vi "update states from tdms.vi"(8 "error in (no error)":errorcluster, 10 "frot panel referances":T1, 11 "p2p vst in":refnum<class "p2p vst.lvclass">) -> (0 "error out":errorcluster, 2 "tdms file mode":T2=enum."P2P - VST", 3 "p2p vst out":refnum<class "p2p vst.lvclass">)   [LabVIEW 2021, in "p2p vst.lvclass"]
uses:
  p2p vst.lvclass
  p2p vst.lvclass/p2p vst.ctl
  device_type/device_type.lvclass
  pulse_tx_vis/device_mode.ctl
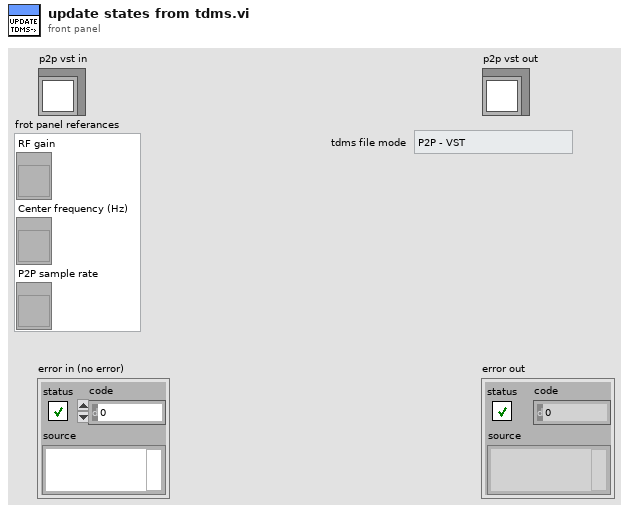
[diagram p1: front panel]
types:
  T1 = cluster{"RF gain ":refnum<vi>, "Center frequency (Hz) ":refnum<vi>, "P2P sample rate":refnum<vi>}
  T2 = typedef "device_mode.ctl" = enum16{"USRP - 180MHz", "5785 - 2*180MHz", "5785 - 3.2GHz", "P2P - VST"}
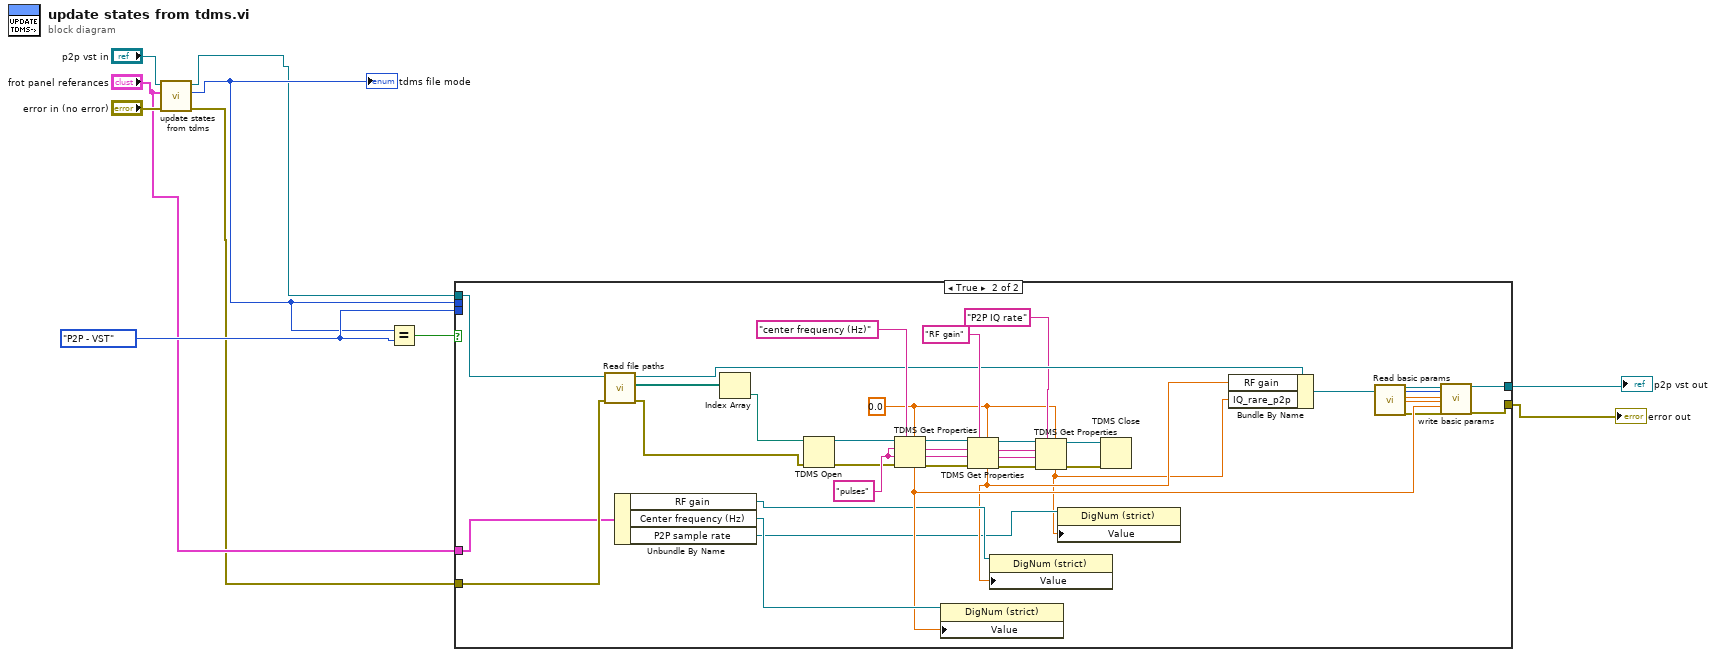
[diagram p0: block diagram]
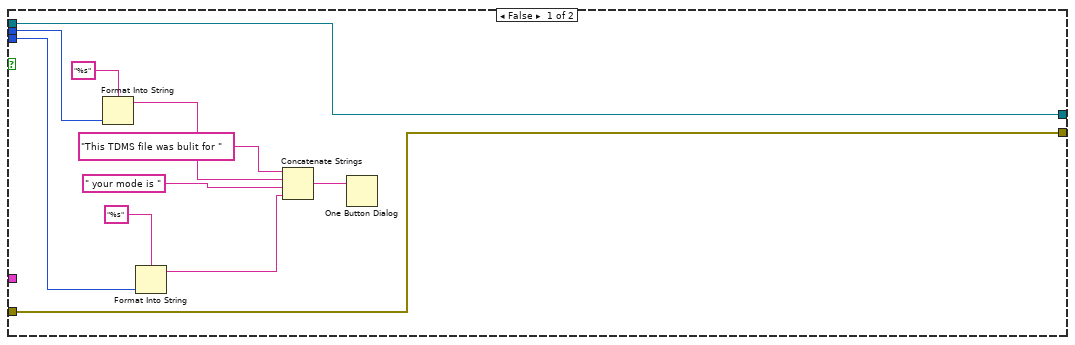
[diagram p2: hidden frame]
diagram:
  w7 = device_mode."P2P - VST" ("Mode")
  n1 = call-parent "update states from tdms.vi"("error in (no error)"="error in (no error)", "frot panel referances"="frot panel referances", "device_type in"="p2p vst in") -> ("error out"=w5:errorcluster, "tdms file mode"=w4:T2, "device_type out"=w3:refnum<class "p2p vst.lvclass">)  [unwired: 6 in]
  "tdms file mode" <- w4
  n2 = Equal?(x=w4, y=w7) -> (x = y?=w8:bool)
  n3 = case shown="True" w8 {
    tunnel: w4 -> [w20 _]
    tunnel: w7 -> [w15 _]
    tunnel: w5 -> [w11 w54]
    tunnel: w3 -> [w12 w52]
    tunnel: "frot panel referances" -> [_ w50]
    tunnel: [w12 w42] -> w1
    tunnel: [w11 w41] -> w2
    frame False {
      n4 = Format Into String(format string="%s", w20) -> (resulting string=w19:string)  [unwired: 2 in, 1 out]
      n5 = Format Into String(format string="%s", w15) -> (resulting string=w14:string)  [unwired: 2 in, 1 out]
      n6 = Concatenate Strings("This TDMS file was bulit for " ("string"), w19, " your mode is " ("string"), w14) -> (w13:string)
      n7 = One Button Dialog(message=w13) -> ()  [unwired: 1 in, 1 out]
    }
    frame True {
      w24 = 0.0
      w59 = "pulses" ("channel name")
      n8 = call-dynamic "Read file paths.vi"("error in (no error)"=w54, "device_type in"=w52) -> ("error out"=w55:errorcluster, "file paths"=w53:path[], "device_type out"=w34:refnum<class "p2p vst.lvclass">)  [unwired: 7 in]
      n9 = Unbundle By Name(w50) -> ("RF gain"=w35:refnum<vi>, "Center frequency (Hz)"=w49:refnum<vi>, "P2P sample rate"=w23:refnum<vi>)
      n10 = Index Array(array=w53) -> (element=w56:path)  [unwired: 1 in]
      n11 = TDMS Open(8:w55, 11:w56) -> (0:w57:errorcluster, 3:w58:refnum<k34>)  [unwired: 5 in]
      n12 = TDMS Get Properties(5:w24, 7:"center frequency (Hz)", 8:w57, 9:w59, 10:w59, 11:w58) -> (0:w37:errorcluster, 1:w38:string, 2:w39:string, 3:w40:refnum<k34>, 4:w44:dbl)  [unwired: 1 out]
      n13 = property class="DigNum (strict)"(reference=w49, "Value"=w44) -> ()  [unwired: 1 in, 2 out]
      n14 = TDMS Get Properties(5:w24, 7:"RF gain", 8:w37, 9:w38, 10:w39, 11:w40) -> (0:w28:errorcluster, 1:w29:string, 2:w30:string, 3:w31:refnum<k34>, 4:w33:dbl)  [unwired: 1 out]
      n15 = property class="DigNum (strict)"(reference=w35, "Value"=w33) -> ()  [unwired: 1 in, 2 out]
      n16 = TDMS Get Properties(5:w24, 7:"P2P IQ rate", 8:w28, 9:w29, 10:w30, 11:w31) -> (0:w27:errorcluster, 3:w26:refnum<k34>, 4:w22:dbl)  [unwired: 3 out]
      n17 = property class="DigNum (strict)"(reference=w23, "Value"=w22) -> ()  [unwired: 1 in, 2 out]
      n18 = TDMS Close(8:w27, 11:w26) -> ()  [unwired: 2 out]
      n19 = Bundle By Name(cluster=w34, "RF gain"=w33, "IQ_rare_p2p"=w22) -> (w32:refnum<class "p2p vst.lvclass">)
      n20 = call-dynamic "Read basic params.vi"("device_type in"=w32) -> ("device_type out"=w48:refnum<class "p2p vst.lvclass">, "buffer size"=w47:u32, "Fs  FPGA"=w46:dbl, "SPC"=w45:dbl, "error out"=w43:errorcluster)  [unwired: 13 in, 1 out]
      n21 = call-dynamic "write basic params.vi"("device_type in"=w48, "buffer size"=w47, "Fs  FPGA"=w46, "SPC"=w45, "center frequency (Hz)"=w44, "error in (no error)"=w43) -> ("device_type out"=w42:refnum<class "p2p vst.lvclass">, "error out"=w41:errorcluster)  [unwired: 12 in]
    }
  }
  "error out" <- w2
  "p2p vst out" <- w1
